vi "SutterController.vi"() -> ()   [LabVIEW 2013]
uses:
  <vilib>/Math Plots/3D Math Plots/3D Scatter/3D Scatter XCtrl/3D Scatter.xctl
  SerialController/Serial Controller.lvclass
  Joystick/Joystick.lvclass
  <vilib>/Utility/file.llb/Read From Spreadsheet File (DBL).vi
  <vilib>/Utility/file.llb/Write To Spreadsheet File (DBL).vi
panel:
  out "element 3":dbl
  out "element 2":dbl
  out "element":dbl
  out "Numeric":i32
  out "TargetPosition":dbl[](array[numeric])
  in  "Manual Pos":bool
  out "data out":string
  in  "Send":bool
  in  "Target Shift":dbl[](array[numeric])=[0.0, 0.0, 0.0]
  in  "stop":bool
  in  "Master":bool
  in  "Set Center":bool
  out "error out":errorcluster
  in  "Z limit":bool
  in  "TopLens":bool
  in  "overide":bool
  out "Range Err":bool
  in  "Set Maximum":bool
  in  "Set Minimum":bool
  out "positionLimits":dbl[][](array[numeric])
  out "Coarse":bool
  out "Locked":bool
  out "AxisStep":dbl[](array[numeric])
  out "ExternalInput":bool
  out "Moving":bool
  in  "Current Position":dbl[](array[numeric])
  out "3D Scatter":refnum<class "3D Plot Datatype.lvclass">[](xcontrol)
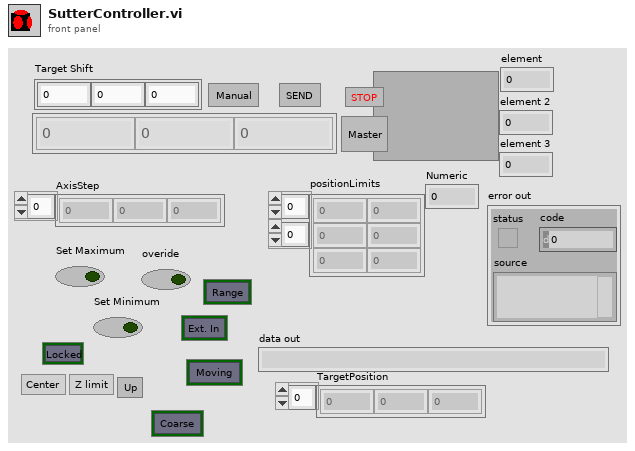
[diagram p1: front panel]
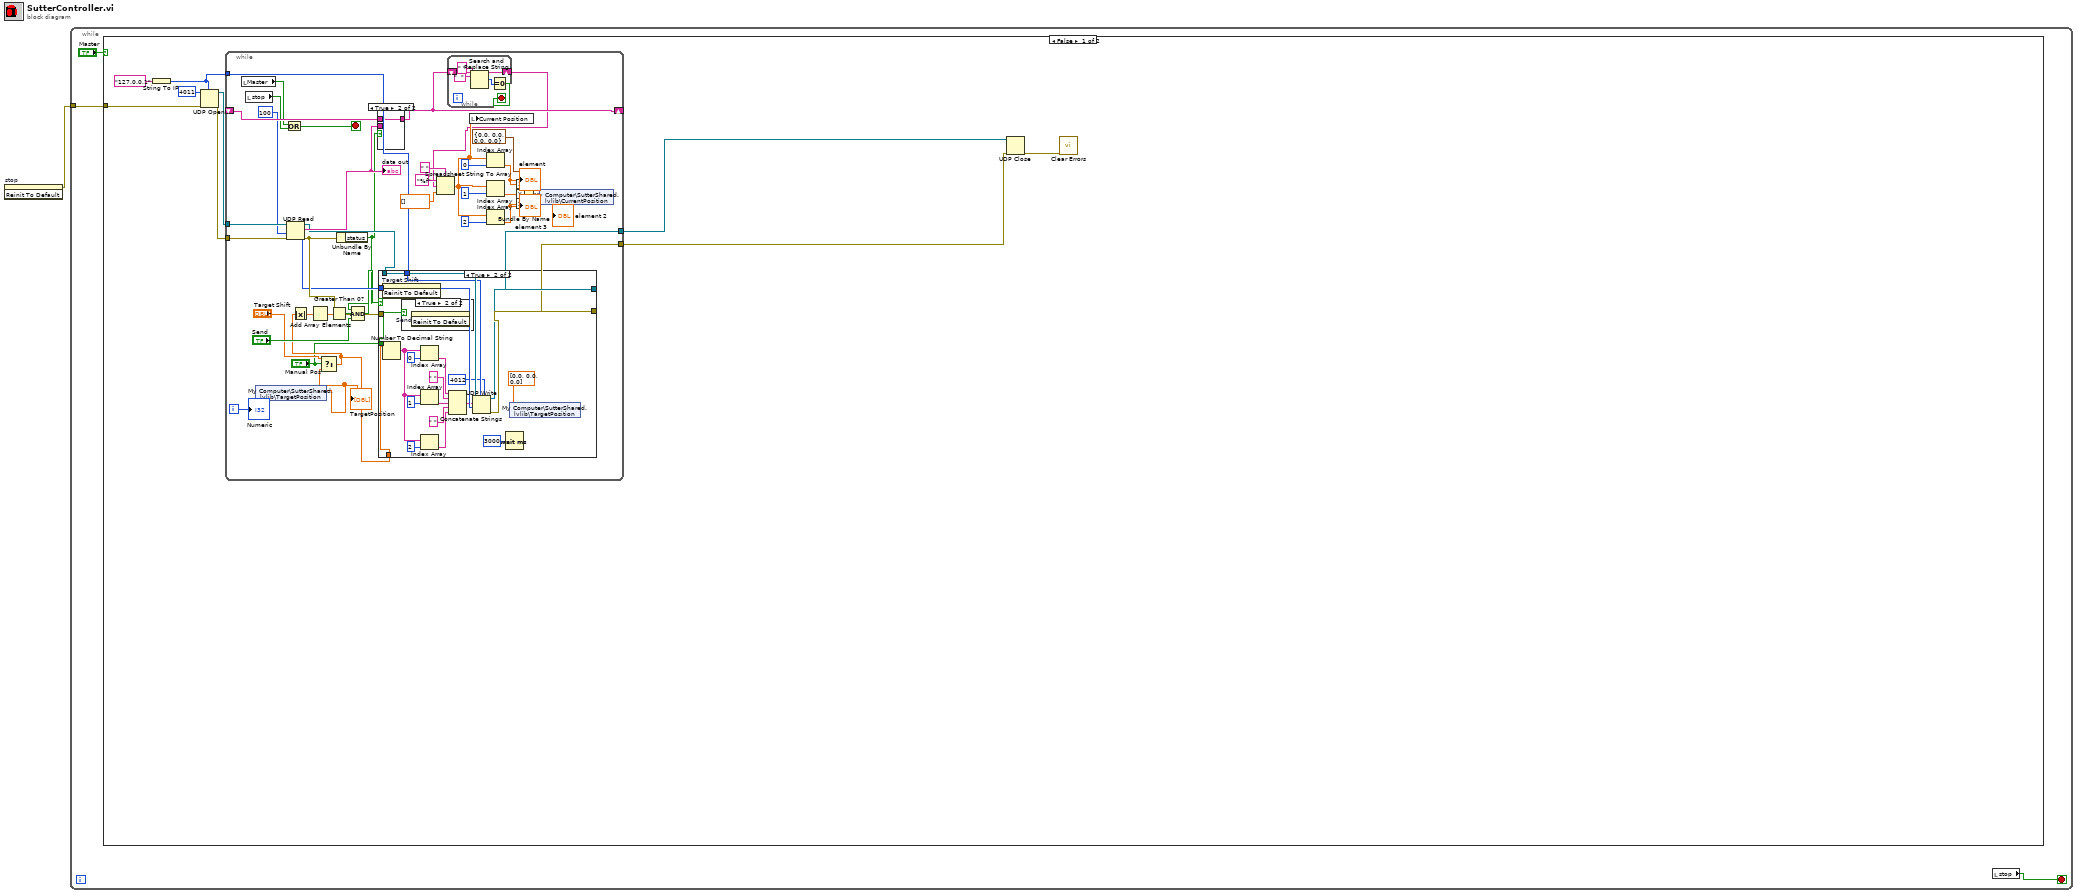
[diagram p0: block diagram]
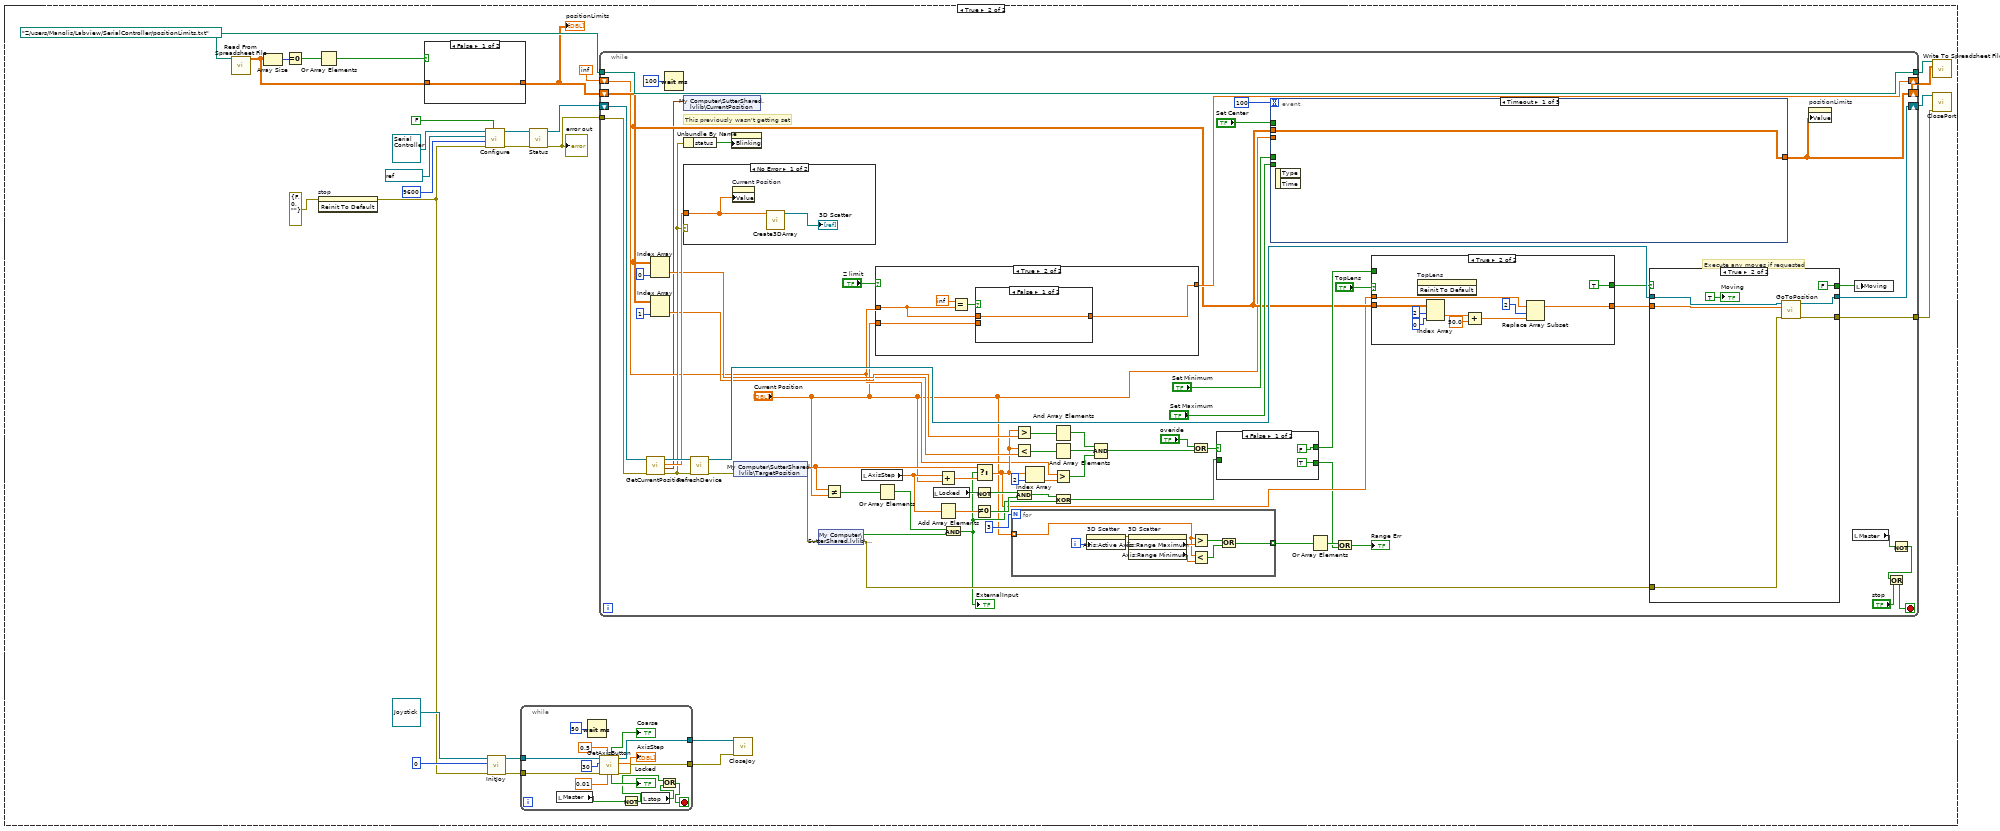
[diagram p5: hidden frame]
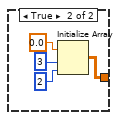
[diagram p6: hidden frame]
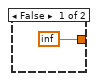
[diagram p7: hidden frame]
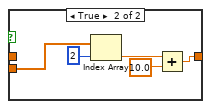
[diagram p8: hidden frame]
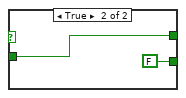
[diagram p10: hidden frame]
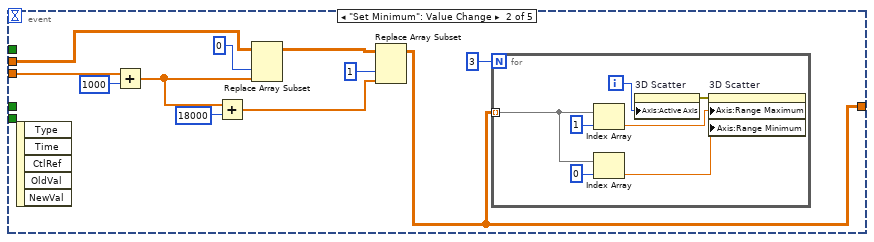
[diagram p11: hidden frame]
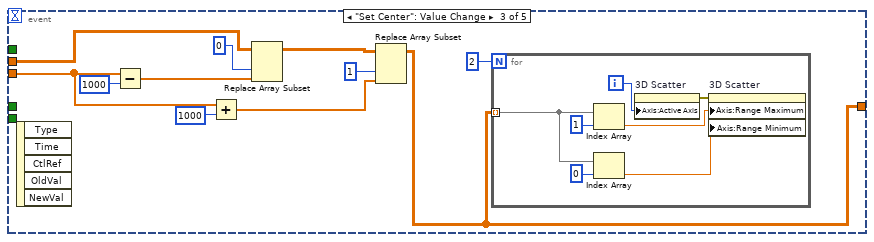
[diagram p12: hidden frame]
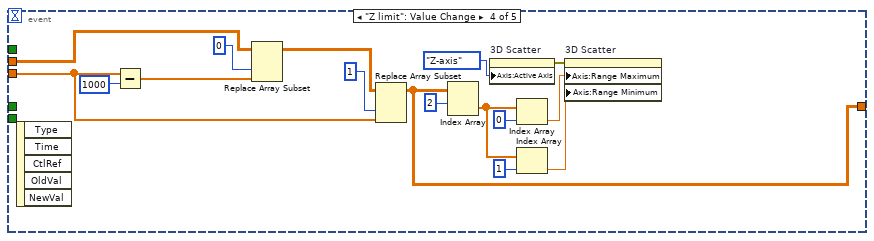
[diagram p13: hidden frame]
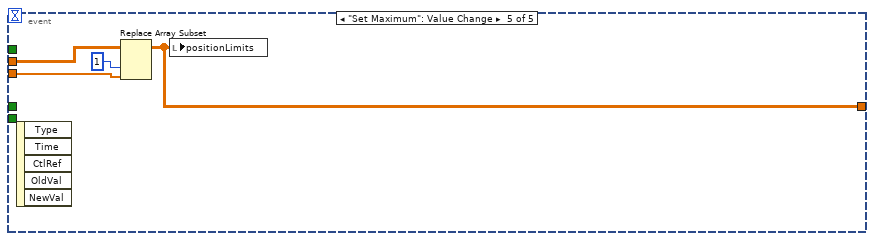
[diagram p14: hidden frame]
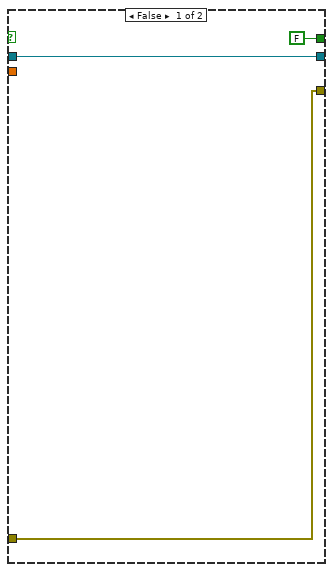
[diagram p15: hidden frame]
diagram:
  n1 = invoke on="stop" class="Bool (strict)" method="Reinit To Default"() -> (error out=w1:errorcluster)  [unwired: 3 in, 2 out]
  n2 = while {
    tunnel: w1 -> [w2]
    stop <- w3 stop-if-true
    n3 = case shown="False" "Master" {
      tunnel: w2 -> [w7 _]
      frame False {
        n4 = String To IP(1:"127.0.0.1" ("name")) -> (0:w6:u32)
        n5 = UDP Open(7:w6, 8:w7, 11:u16 4011 ("port")) -> (port=w9:refnum<k16>, 0:w12:errorcluster)  [unwired: 2 in, 1 out]
        n6 = while {
          tunnel: w9 -> [w51]
          tunnel: [w31] -> w10
          shift-right: [w15] -> _
          shift-left: _ -> [w49]
          tunnel: w12 -> [w48]
          tunnel: [w29] -> w13
          tunnel: w6 -> [w21]
          i -> [w17]
          stop <- w35 stop-if-true
          w28 = 100 ("timeout ms (25000)")
          n7 = local read "Master"() -> (w34:bool)
          n8 = local read "stop"() -> (w36:bool)
          n9 = shared-variable "My Computer\\SutterShared.lvlib\\TargetPosition"() -> (w16:dbl[])  [unwired: 1 in, 1 out]
          "TargetPosition" <- w16
          n10 = Or(x=w34, y=w36) -> (x .or. y?=w35:bool)
          n11 = UDP Read(connection ID=w51, timeout ms (25000)=w28, 8:w48) -> (data out=w50:string, error out=w30:errorcluster, 3:w32:refnum<k16>)  [unwired: 1 in, 2 out]
          "data out" <- w50
          n12 = Select(t="Target Shift", s="Manual Pos", f=w16) -> (s? t:f=w19:dbl[])
          n13 = Absolute Value(x=w19) -> (abs(x)=w25:dbl[])
          n14 = Add Array Elements(numeric array=w25) -> (sum=w24:dbl)
          n15 = Greater Than 0?(x=w24) -> (x > 0?=w23:bool)
          n16 = Unbundle By Name(w30) -> ("status"=w26:bool)
          n17 = Compound Arithmetic op=AND(w26, w23, "Send") -> (w27:bool)
          n18 = case shown="True" w26 {
            tunnel: w50 -> [w80 _]
            tunnel: [w80 w81] -> w15
            tunnel: w49 -> [_ w81]
            frame False {
            }
            frame True {
            }
          }
          n19 = case shown="True" w27 {
            tunnel: w32 -> [w59 w78]
            tunnel: [w59 w77] -> w31
            tunnel: w30 -> [w58 _]
            tunnel: [w58 w79] -> w29
            tunnel: w28 -> [_ w76]
            tunnel: w19 -> [_ w75]
            tunnel: w21 -> [_ w65]
            tunnel: "Manual Pos" -> [_ w61]
            frame False {
            }
            frame True {
              n20 = Number To Decimal String(number=w75) -> (decimal integer string=w73:string[])  [unwired: 1 in]
              n21 = invoke on="Target Shift" class="Arr (strict)" method="Reinit To Default"() -> ()  [unwired: 3 in, 3 out]
              n22 = case shown="True" w61 {
                frame False {
                }
                frame True {
                  n23 = invoke on="Send" class="Bool (strict)" method="Reinit To Default"() -> ()  [unwired: 3 in, 3 out]
                }
              }
              n24 = Index Array(array=w73, index=0) -> (element=w74:string)
              n25 = Index Array(array=w73, index=1) -> (element=w69:string)
              n26 = Index Array(array=w73, index=2) -> (element=w68:string)
              n27 = Concatenate Strings(w74, " " ("string"), w69, " " ("string"), w68) -> (w63:string)
              n28 = UDP Write(address=w65, port or service name=u16 4012, connection ID=w78, data in=w63, 9:w76) -> (error out=w79:errorcluster, 3:w77:refnum<k16>)  [unwired: 1 in]
              n29 = Wait (ms)(milliseconds to wait=u32 3000) -> ()  [unwired: 1 out]
              n30 = shared-variable "My Computer\\SutterShared.lvlib\\TargetPosition"(dbl[] [0.0, 0.0, 0.0] ("TargetPosition")) -> ()  [unwired: 1 in, 1 out]
            }
          }
          n31 = while {
            shift-right: [w52] -> w14
            shift-left: w15 -> [w57]
            stop <- w54 stop-if-true
            n32 = Search and Replace String(input string=w57, search string="  ", replace string=" " ("replace string (\"\")")) -> (result string=w52:string, number of replacements=w53:i32)  [unwired: 5 in, 2 out]
            n33 = Equal To 0?(x=w53) -> (x = 0?=w54:bool)
          }
          n34 = Spreadsheet String To Array(delimiter (Tab)=" ", format string="%f", spreadsheet string=w14, array type (2D Dbl)=dbl[] []) -> (array=w33:dbl[])
          n35 = local write "Current Position"(w33) -> ()
          n36 = Index Array(array=w33, index=0) -> (element=w45:dbl)
          "element" <- w45
          n37 = Index Array(array=w33, index=1) -> (element=w44:dbl)
          "element 2" <- w44
          n38 = Index Array(array=w33, index=2) -> (element=w43:dbl)
          "element 3" <- w43
          n39 = Bundle By Name(cluster=cluster{"X":dbl, "Y":dbl, "Z":dbl, "Depth":dbl} {"X"=0.0, "Y"=0.0, "Z"=0.0, "Depth"=0.0}, "X"=w45, "Y"=w44, "Z"=w43) -> (w47:cluster{"X":dbl, "Y":dbl, "Z":dbl, "Depth":dbl})
          n40 = shared-variable "My Computer\\SutterShared.lvlib\\CurrentPosition"(w47) -> ()  [unwired: 1 in, 1 out]
          "Numeric" <- w17
        }
        n41 = UDP Close(connection ID=w10, 8:w13) -> (error out=w8:errorcluster)  [unwired: 1 out]
        n42 = call <vilib>:"Clear Errors.vi"("error in (no error)"=w8) -> ()  [unwired: 6 in, 1 out]
      }
      frame True {
        w92 = path "Z:/users/Manolis/Labview/SerialController/positionLimits.txt" ("Path")
        n43 = call-poly <vilib>:"Read From Spreadsheet File.vi"("file path (dialog if empty)"=w92) -> ("all rows"=w87:dbl[][])  [unwired: 6 in, 4 out]
        n44 = Array Size(array=w87) -> (size(s)=w89:i32[])
        n45 = Equal To 0?(x=w89) -> (x = 0?=w88:bool[])
        n46 = invoke on="stop" class="Bool (strict)" method="Reinit To Default"(error in=errorcluster {"status"=FALSE, "code"=0, "source"=""} ("error in (no error)")) -> (error out=w93:errorcluster)  [unwired: 2 in, 2 out]
        n47 = Or Array Elements(Boolean array=w88) -> (logical OR=w85:bool)
        n48 = case shown="False" w85 {
          tunnel: w87 -> [w109 _]
          tunnel: [w109 w110] -> w86
          frame False {
          }
          frame True {
            n49 = Initialize Array(0.0 ("element"), 3 ("dimension size"), 2 ("dimension size")) -> (w110:dbl[][])
          }
        }
        "positionLimits" <- w86
        n50 = call-dynamic "Configure.vi"("Reset"=FALSE, "error in (no error)"=w93, "baud rate (9600)"=u32 9600, "VISA resource name"=refnum<visa-resource-name> "COM3", "Serial Controller in"=refnum<class "Serial Controller.lvclass"> refnum) -> ("error out"=w107:errorcluster, "Serial Controller out"=w108:refnum<class "Serial Controller.lvclass">)  [unwired: 5 in]
        n51 = call-dynamic "InitJoy.vi"("error in (no error)"=w93, "device index"=0, "Joystick in"=refnum<class "Joystick.lvclass"> refnum) -> ("error out"=w97:errorcluster, "Joystick out"=w98:refnum<class "Joystick.lvclass">)  [unwired: 7 in]
        n52 = while {
          tunnel: w98 -> [w127]
          tunnel: w97 -> [w126]
          tunnel: [w121] -> w96
          tunnel: [w122] -> w95
          stop <- w116 stop-if-true
          n53 = local read "Master"() -> (w115:bool)
          n54 = Wait (ms)(milliseconds to wait=u32 50) -> ()  [unwired: 1 out]
          n55 = call-dynamic "GetAxisButton.vi"("coarseFactor"=0.01, "fastFactor"=0.5, "error in (no error)"=w126, "timeout(s)"=u32 30, "Joystick in"=w127) -> ("error out"=w122:errorcluster, "AxisStep"=→"AxisStep":dbl[], "Joystick out"=w121:refnum<class "Joystick.lvclass">, "lock"=→"Locked":bool, "Coarse"=→"Coarse":bool)  [unwired: 2 in]
          n56 = Not(x=w115) -> (.not. x?=w114:bool)
          n57 = local read "stop"() -> (w117:bool)
          n58 = Or(x=w114, y=w117) -> (x .or. y?=w116:bool)
        }
        n59 = call-dynamic "Status.vi"("error in (no error)"=w107, "Serial Controller in"=w108) -> ("error out"=w82:errorcluster, "Serial Controller out"=w83:refnum<class "Serial Controller.lvclass">)  [unwired: 7 in, 1 out]
        "error out" <- w82
        n60 = while {
          shift-right: [w187] -> w102
          shift-left: w83 -> [w195]
          tunnel: [w176] -> w101
          tunnel: w82 -> [w182]
          tunnel: w92 -> [w167]
          tunnel: [w167] -> w91
          shift-right: [w153] -> w90
          shift-left: w86 -> [w150]
          shift-right: [w151] -> _
          shift-left: inf -> [w147]
          stop <- w131 stop-if-true
          # "Execute any moves if requested"
          # "This previously wasn't getting set"
          n61 = call-dynamic "GetCurrentPosition.vi"("error in (no error)"=w182, "Serial Controller in"=w195) -> ("error out"=w191:errorcluster, "PositionBundle"=w141:cluster{"X":dbl, "Y":dbl, "Z":dbl, "Depth":dbl}, "Position"=w192:dbl[], "Serial Controller out"=w193:refnum<class "Serial Controller.lvclass">)  [unwired: 6 in]
          n62 = Index Array(array=w150, index (col)=0 ("disabled index (col)")) -> (element=w166:dbl[])  [unwired: 1 in]
          n63 = Index Array(array=w150, index (col)=1 ("disabled index (col)")) -> (element=w165:dbl[])  [unwired: 1 in]
          n64 = Wait (ms)(milliseconds to wait=u32 100) -> ()  [unwired: 1 out]
          n65 = shared-variable "My Computer\\SutterShared.lvlib\\CurrentPosition"(w141) -> ()  [unwired: 1 in, 1 out]
          n66 = Unbundle By Name(w191) -> ("status"=w190:bool)
          n67 = case shown="No Error" w191 {
            tunnel: w192 -> [w299 _]
            frame No Error {
              n68 = property on="Current Position" class="Arr (strict)"("Value"=w299) -> ()  [unwired: 2 in, 2 out]
              n69 = call "Create3DArray.vi"("Position"=w299) -> ("3D Plot lvclass Array out"=→"3D Scatter":refnum<class "3D Plot Datatype.lvclass">[])  [unwired: 10 in]
            }
            frame Error {
            }
          }
          n70 = call-dynamic "RefreshDevice.vi"("error in (no error)"=w191, "Serial Controller in"=w193) -> ("error out"=w181:errorcluster, "Serial Controller out"=w183:refnum<class "Serial Controller.lvclass">)  [unwired: 8 in]
          n71 = property on="Current Position" class="Arr (strict)"("Blinking"=w190) -> ()  [unwired: 2 in, 2 out]
          n72 = shared-variable "My Computer\\SutterShared.lvlib\\TargetPosition"(error in=w181) -> (w179:dbl[], error out=w175:errorcluster)
          n73 = shared-variable "My Computer\\SutterShared.lvlib\\Move"(error in=w175) -> (w172:bool, error out=w174:errorcluster)
          n74 = Not Equal?(x=w179, y="Current Position") -> (x != y?=w180:bool[])
          n75 = local read "AxisStep"() -> (w189:dbl[])
          n76 = case shown="True" "Z limit" {
            tunnel: w147 -> [_ w205]
            tunnel: [inf w208] -> w151
            tunnel: "Current Position" -> [_ w209]
            frame False {
            }
            frame True {
              n77 = Equal?(x=inf, y=w205) -> (x = y?=w206:bool)
              n78 = case shown="False" w206 {
                tunnel: w209 -> [_ w215]
                tunnel: [w210 w212] -> w208
                tunnel: w205 -> [w210 _]
                frame False {
                }
                frame True {
                  n79 = Index Array(array=w215, index=2) -> (element=w213:dbl)
                  n80 = Add(x=w213, y=10.0) -> (x+y=w212:dbl)
                }
              }
            }
          }
          n81 = Or Array Elements(Boolean array=w180) -> (logical OR=w173:bool)
          n82 = local read "Locked"() -> (w185:bool)
          n83 = Add(x=w189, y="Current Position") -> (x+y=w178:dbl[])
          n84 = Add Array Elements(numeric array=w189) -> (sum=w188:dbl)
          n85 = And(x=w173, y=w172) -> (x .and. y?=w171:bool)
          "ExternalInput" <- w171
          n86 = Not(x=w185) -> (.not. x?=w184:bool)
          n87 = Not Equal To 0?(x=w188) -> (x != 0?=w186:bool)
          n88 = Select(t=w179, s=w171, f=w178) -> (s? t:f=w149:dbl[])
          n89 = for {
            N: 3 -> [_]
            tunnel: "Current Position" -> [w199] mode=indexing
            tunnel: [w196] -> w136 mode=indexing
            i -> [w202]
            n90 = property on="3D Scatter" class="3D Scatter (strict)"("Axis:Active Axis"=w202) -> (error out=w203:errorcluster)  [unwired: 2 in, 1 out]
            n91 = property on="3D Scatter" class="3D Scatter (strict)"(error in=w203) -> ("Axis:Range Maximum"=w200:sgl, "Axis:Range Minimum"=w201:sgl)  [unwired: 1 in, 2 out]
            n92 = Greater?(x=w199, y=w200) -> (0:w198:bool)
            n93 = Less?(x=w199, y=w201) -> (x < y?=w197:bool)
            n94 = Or(x=w198, y=w197) -> (x .or. y?=w196:bool)
          }
          n95 = Greater?(x=w149, y=w166) -> (0:w162:bool[])
          n96 = Less?(x=w149, y=w165) -> (x < y?=w161:bool[])
          n97 = And(x=w184, y=w186) -> (x .and. y?=w177:bool)
          n98 = Index Array(array=w149, index=2) -> (element=w146:dbl)
          n99 = And Array Elements(Boolean array=w162) -> (logical AND=w145:bool)
          n100 = And Array Elements(Boolean array=w161) -> (logical AND=w144:bool)
          n101 = Greater?(x=w147, y=w146) -> (0:w142:bool)
          n102 = Exclusive Or(1:w171, 2:w177) -> (0:w160:bool)
          n103 = Compound Arithmetic op=AND(w145, w144, w142) -> (w143:bool)
          n104 = Or(x="overide", y=w143) -> (x .or. y?=w159:bool)
          n105 = case shown="False" w159 {
            tunnel: w160 -> [_ w231]
            tunnel: [FALSE w231] -> w156
            tunnel: [TRUE FALSE] -> w133
            frame False {
            }
            frame True {
            }
          }
          n106 = event shown="[0] Timeout" {
            selector: _ -> [_ _ _ _ _]
            dyn-events: _ -> [_ _ _ _ _]
            timeout: 100 -> [_ _ _ _ _]
            tunnel: "Set Minimum" -> [_ _ _ _ _]
            tunnel: "Current Position" -> [_ w241 w251 w278 w288]
            tunnel: w150 -> [w232 w243 w253 w279 w287]
            tunnel: "Set Maximum" -> [_ _ _ _ _]
            tunnel: [w232 w233 w252 w276 w285] -> w153
            tunnel: "Set Center" -> [_ _ _ _ _]
            event Timeout {
              n107 = event-data() -> ()  [unwired: 1 in, 2 out]
            }
            event "Set Minimum": Value Change {
              n108 = event-data() -> ()  [unwired: 1 in, 5 out]
              n109 = Add(x=w241, y=1000) -> (x+y=w237:dbl[])
              n110 = Add(x=w237, y=18000) -> (x+y=w236:dbl[])
              n111 = Replace Array Subset(array=w243, new element=w237, index (col)=0 ("disabled index (col)")) -> (w238:dbl[][])  [unwired: 1 in]
              n112 = Replace Array Subset(array=w238, new element=w236, index (col)=1 ("disabled index (col)")) -> (w233:dbl[][])  [unwired: 1 in]
              n113 = for {
                N: 3 -> [_]
                tunnel: w233 -> [w249] mode=indexing
                i -> [w250]
                n114 = Index Array(array=w249, index=1) -> (element=w247:dbl)
                n115 = Index Array(array=w249, index=0) -> (element=w248:dbl)
                n116 = property on="3D Scatter" class="3D Scatter (strict)"("Axis:Active Axis"=w250) -> (error out=w244:errorcluster)  [unwired: 2 in, 1 out]
                n117 = property on="3D Scatter" class="3D Scatter (strict)"(error in=w244, "Axis:Range Maximum"=w247, "Axis:Range Minimum"=w248) -> ()  [unwired: 1 in, 2 out]
              }
            }
            event "Set Center": Value Change {
              n118 = event-data() -> ()  [unwired: 1 in, 5 out]
              n119 = Subtract(x=w251, y=1000) -> (x-y=w257:dbl[])
              n120 = Add(x=w251, y=1000) -> (x+y=w256:dbl[])
              n121 = Replace Array Subset(array=w253, new element=w257, index (col)=0 ("disabled index (col)")) -> (w258:dbl[][])  [unwired: 1 in]
              n122 = Replace Array Subset(array=w258, new element=w256, index (col)=1 ("disabled index (col)")) -> (w252:dbl[][])  [unwired: 1 in]
              n123 = for {
                N: 2 -> [_]
                tunnel: w252 -> [w267] mode=indexing
                i -> [w268]
                n124 = Index Array(array=w267, index=1) -> (element=w265:dbl)
                n125 = Index Array(array=w267, index=0) -> (element=w266:dbl)
                n126 = property on="3D Scatter" class="3D Scatter (strict)"("Axis:Active Axis"=w268) -> (error out=w262:errorcluster)  [unwired: 2 in, 1 out]
                n127 = property on="3D Scatter" class="3D Scatter (strict)"(error in=w262, "Axis:Range Maximum"=w265, "Axis:Range Minimum"=w266) -> ()  [unwired: 1 in, 2 out]
              }
            }
            event "Z limit": Value Change {
              n128 = event-data() -> ()  [unwired: 1 in, 5 out]
              n129 = Subtract(x=w278, y=1000) -> (x-y=w280:dbl[])
              n130 = Replace Array Subset(array=w279, new element=w280, index (col)=0 ("disabled index (col)")) -> (w281:dbl[][])  [unwired: 1 in]
              n131 = Replace Array Subset(array=w281, new element=w278, index (col)=1 ("disabled index (col)")) -> (w276:dbl[][])  [unwired: 1 in]
              n132 = Index Array(array=w276, index (row)=2) -> (element=w271:dbl[])  [unwired: 1 in]
              n133 = property on="3D Scatter" class="3D Scatter (strict)"("Axis:Active Axis"=enum16{"X-axis", "Y-axis", "Z-axis"}."Z-axis") -> (error out=w277:errorcluster)  [unwired: 2 in, 1 out]
              n134 = Index Array(array=w271, index=0) -> (element=w270:dbl)
              n135 = Index Array(array=w271, index=1) -> (element=w269:dbl)
              n136 = property on="3D Scatter" class="3D Scatter (strict)"(error in=w277, "Axis:Range Maximum"=w270, "Axis:Range Minimum"=w269) -> ()  [unwired: 1 in, 2 out]
            }
            event "Set Maximum": Value Change {
              n137 = event-data() -> ()  [unwired: 1 in, 5 out]
              n138 = Replace Array Subset(array=w287, new element=w288, index (col)=1 ("disabled index (col)")) -> (w285:dbl[][])  [unwired: 1 in]
              n139 = local write "positionLimits"(w285) -> ()
            }
          }
          n140 = Or Array Elements(Boolean array=w136) -> (logical OR=w134:bool)
          n141 = Or(x=w134, y=w133) -> (x .or. y?=→"Range Err":bool)
          n142 = case shown="True" "TopLens" {
            tunnel: w156 -> [w217 _]
            tunnel: [w217 TRUE] -> w155
            tunnel: w149 -> [w216 w226]
            tunnel: [w216 w224] -> w154
            tunnel: w150 -> [_ w223]
            frame False {
            }
            frame True {
              n143 = invoke on="TopLens" class="Bool (strict)" method="Reinit To Default"() -> ()  [unwired: 3 in, 3 out]
              n144 = Index Array(array=w223, index (row)=2 ("disabled index (row)"), index (col)=0 ("disabled index (col)")) -> (element=w220:dbl)
              n145 = Add(x=w220, y=50.0) -> (x+y=w219:dbl)
              n146 = Replace Array Subset(array=w226, new element=w219, index=2) -> (w224:dbl[])
            }
          }
          n147 = case shown="True" w155 {
            tunnel: w183 -> [w291 w298]
            tunnel: [w291 w294] -> w187
            tunnel: w174 -> [w290 w297]
            tunnel: [w290 w293] -> w176
            tunnel: w154 -> [_ w296]
            tunnel: [FALSE FALSE] -> w140
            frame False {
            }
            frame True {
              n148 = call-dynamic "GoToPosition.vi"("error in (no error)"=w297, "Position"=w296, "Serial Controller in"=w298) -> ("error out"=w293:errorcluster, "Serial Controller out"=w294:refnum<class "Serial Controller.lvclass">)  [unwired: 6 in, 1 out]
              "Moving" <- TRUE ("Boolean")
            }
          }
          n149 = property on="positionLimits" class="Arr (strict)"("Value"=w153) -> ()  [unwired: 2 in, 2 out]
          n150 = local read "Master"() -> (w130:bool)
          n151 = local write "Moving"(w140) -> ()
          n152 = Not(x=w130) -> (.not. x?=w129:bool)
          n153 = Or(x=w129, y="stop") -> (x .or. y?=w131:bool)
        }
        n154 = call-dynamic "CloseJoy.vi"("error in (no error)"=w95, "Joystick in"=w96) -> ()  [unwired: 9 in, 1 out]
        n155 = call-poly <vilib>:"Write To Spreadsheet File.vi"("2D data"=w90, "file path (dialog if empty)"=w91) -> ()  [unwired: 6 in, 1 out]
        n156 = call-dynamic "ClosePort.vi"("error in (no error)"=w101, "Serial Controller in"=w102) -> ()  [unwired: 9 in, 1 out]
      }
    }
    n157 = local read "stop"() -> (w3:bool)
  }
